vi "sutter driver track targ.vi"() -> ()   [LabVIEW 2016]
uses:
  <vilib>/userdefined/High Color/IMAQdx.ctl
  <vilib>/Instr/_visa.llb/VISA Configure Serial Port (Instr).vi
  <vilib>/vision/driver/NI_Vision_Acquisition_Software.lvlib
panel:
  out "Numeric 2":i32
  out "appended array":sgl[][](array[numeric])
  out "output array":dbl[](array[numeric])
  out "error out":errorcluster
  in  "stop":bool
  out "Send Position":dbl[](array[numeric])
  out "Curent Position":dbl[](array[numeric])
  out "Numeric":i32
  in  "VISA resource name":refnum<visa-resource-name>
  out "Pos error":sgl[](array[numeric])
  out "Injector Pos":sgl[](array[numeric])
  out "Coordinates":i32[](array[numeric])
  out "Image":T1(plugin-control)
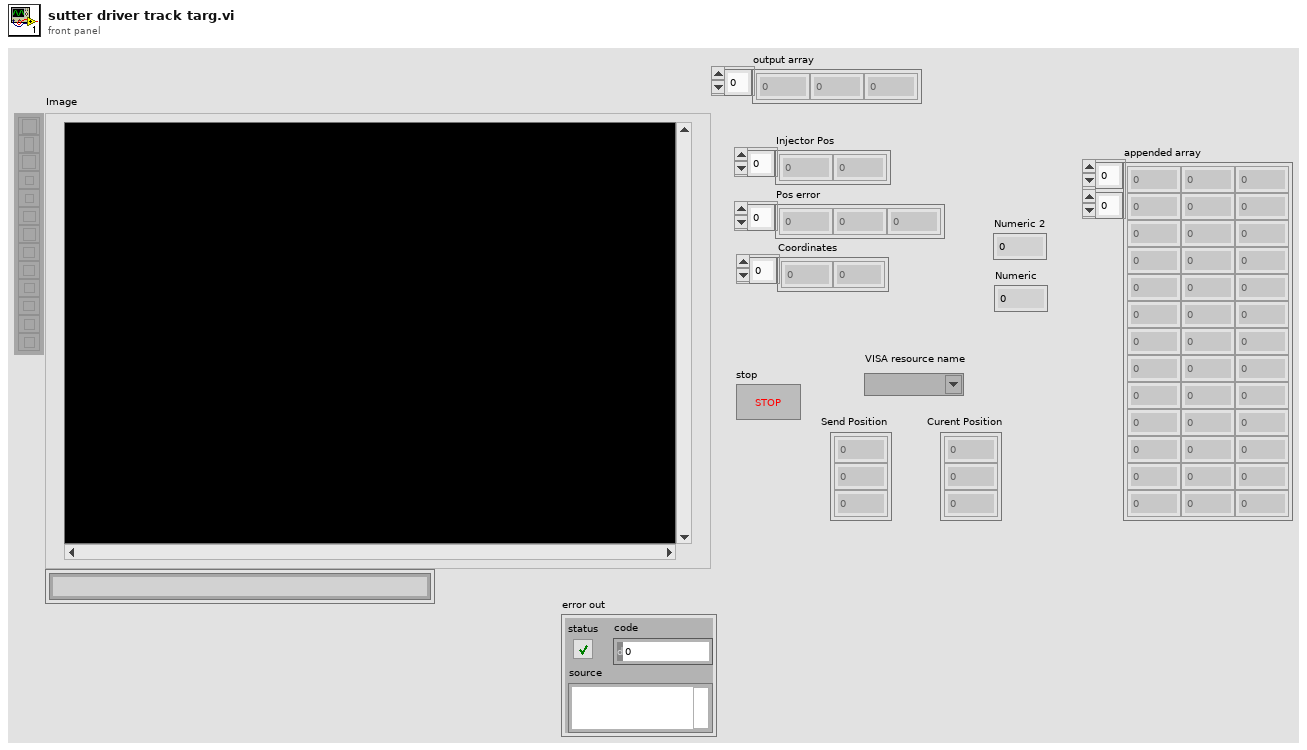
[diagram p1: front panel]
types:
  T1 = typedef "IMAQ Image.ctl" = refnum<image>
  T2 = typedef "IMAQdx.ctl" = refnum<k21>
  T3 = typedef "Image Type" = u32
  T4 = cluster{"Left":i32, "Top":i32, "Right":i32, "Bottom":i32}
  T5 = cluster{"Position":cluster{"x":sgl, "y":sgl}, "Angle":sgl, "Scale":sgl, "Score":sgl, "Bounding Box":cluster{"x":sgl, "y":sgl}[]}[]
  T6 = cluster{"Position":cluster{"x":sgl, "y":sgl}, "Angle":sgl, "Scale":sgl, "Score":sgl, "Bounding Box":cluster{"x":sgl, "y":sgl}[]}
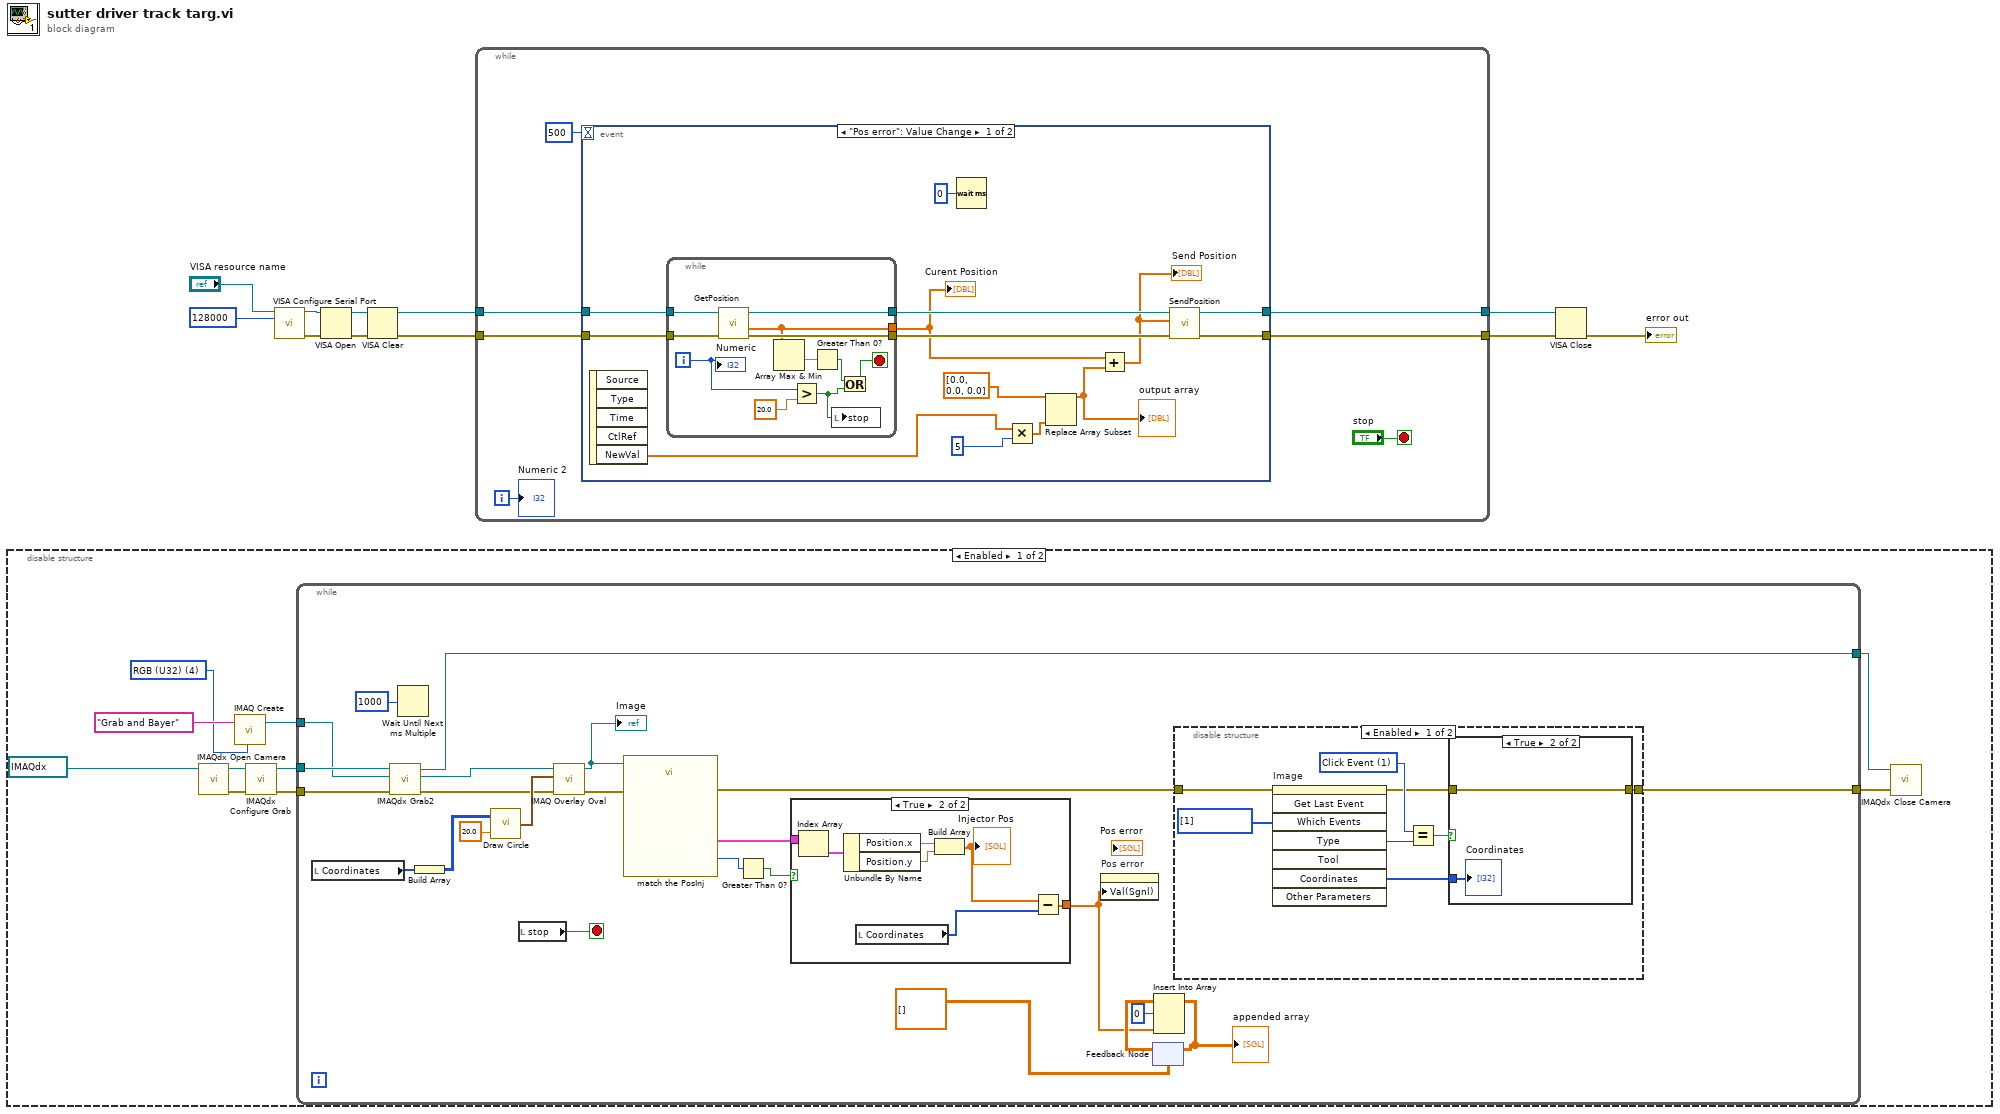
[diagram p0: block diagram]
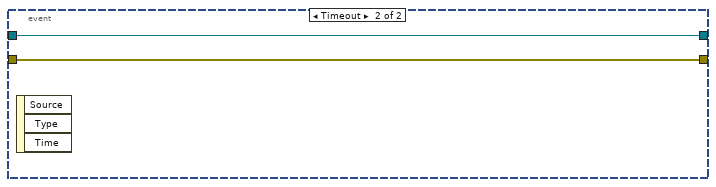
[diagram p2: hidden frame]
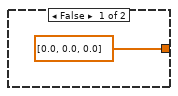
[diagram p3: hidden frame]
diagram:
  n1 = disable-structure shown="Enabled" {
    frame Enabled {
      w14 = T3 4 items=["Grayscale (U8)", "Grayscale (I16)", "Grayscale (SGL)", "Complex (CSG)", "RGB (U32)", "HSL (U32)", "RGB (U64)", "Grayscale (U16)"] ("Image Type")
      n2 = call <vilib>:"IMAQdx Open Camera.vi"("Session In"=T2 "cam1") -> ("error out"=w17:errorcluster, "Session Out"=w18:T2)  [unwired: 2 in, 7 out]
      n3 = call "IMAQ Create"("Image Name"="Grab and Bayer", "Image Type"=w14) -> ("New Image"=w15:T1)  [unwired: 2 in, 2 out]
      n4 = call <vilib>:"IMAQdx Configure Grab.vi"("error in"=w17, "Session In"=w18) -> ("error out"=w20:errorcluster, "Session Out"=w19:T2)  [unwired: 8 out]
      n5 = while {
        tunnel: w15 -> [w43]
        tunnel: w20 -> [w44]
        tunnel: w19 -> [w45]
        tunnel: [w34] -> w13
        tunnel: [w29] -> w12
        stop <- w41 stop-if-true
        n6 = local read "Coordinates"() -> (w40:i32[])
        n7 = call <vilib>:"IMAQdx Grab2.vi"("error in"=w44, "Image In"=w43, "Session In"=w45) -> ("error out"=w35:errorcluster, "Image Out"=w37:T1, "Session Out"=w34:T2)  [unwired: 5 in, 1 out]
        n8 = Wait Until Next ms Multiple(millisecond multiple=u32 1000) -> ()  [unwired: 1 out]
        n9 = Build Array(w40) -> (w39:i32[][])
        n10 = call "Draw Circle.vi"("radius"=20.0, "Pos XY"=w39) -> ("Bound out"=w36:T4)
        n11 = local read "stop"() -> (w41:bool)
        n12 = call "IMAQ Overlay Oval"("error in (no error)"=w35, "Bounding Rectangle"=w36, "Image"=w37) -> ("error out"=w31:errorcluster, "Image Out"=w32:T1)  [unwired: 7 in]
        "Image" <- w32
        n13 = call "match the PosInj"("Image In"=w32, "error in"=w31) -> ("Matches (Pattern Matching 1)"=w33:T5, "Number of Matches (Pattern Matching 1)"=w28:i32, "error out"=w30:errorcluster)  [unwired: 22 in, 1 out]
        n14 = Greater Than 0?(x=w28) -> (x > 0?=w27:bool)
        n15 = case shown="True" w27 {
          tunnel: w33 -> [_ w53]
          tunnel: [sgl[] [0.0, 0.0, 0.0] w47] -> w22
          frame False {
          }
          frame True {
            n16 = Index Array(array=w53) -> (element=w50:T6)  [unwired: 1 in]
            n17 = Unbundle By Name(w50) -> ("Position.x"=w52:sgl, "Position.y"=w51:sgl)
            n18 = local read "Coordinates"() -> (w48:i32[])
            n19 = Build Array(w52, w51) -> (w49:sgl[])
            "Injector Pos" <- w49
            n20 = Subtract(x=w49, y=w48) -> (x-y=w47:sgl[])
          }
        }
        n21 = property on="Pos error" class="Arr (strict)"("Val(Sgnl)"=w22) -> ()  [unwired: 2 in, 2 out]
        n22 = feedback #1(dbl[][] []) -> (w24:dbl[][])
        n23 = Insert Into Array(array=w24, index (row)=0, new element=w22) -> (w26:dbl[][])  [unwired: 1 in]
        "appended array" <- w26
        n24 = feedback-in #1(w26) -> ()
        n25 = disable-structure shown="Enabled" {
          disable-tunnel: [w55 _] -> w29
          disable-tunnel: w30 -> [w54 _]
          frame Enabled {
            w59 = 1 items=["No Event"=0, "Click Event"=1, "Draw Event"=2, "Size Event"=4, "Scroll Event"=5, "Double Click Event"=8]
            w60 = i32[] [1] items=["No Event"=0, "Click Event"=1, "Draw Event"=2, "Size Event"=4, "Scroll Event"=5, "Double Click Event"=8] ("Which Events")
            n26 = invoke on="Image" class="ImageControl" method="Get Last Event"(error in=w54, "Which Events"=w60) -> (error out=w56:errorcluster, "Type"=w58:i32, "Coordinates"=w61:i32[])  [unwired: 6 in, 5 out]
            n27 = Equal?(x=w59, y=w58) -> (x = y?=w57:bool)
            n28 = case shown="True" w57 {
              tunnel: w61 -> [_ w64]
              tunnel: w56 -> [w62 w63]
              tunnel: [w62 w63] -> w55
              frame False {
              }
              frame True {
                "Coordinates" <- w64
              }
            }
          }
          frame Disabled {
          }
        }
      }
      n29 = call <vilib>:"IMAQdx Close Camera.vi"("error in"=w12, "Session In"=w13) -> ()  [unwired: 9 in, 1 out]
    }
    frame Disabled {
    }
  }
  n30 = call-poly "VISA Configure Serial Port"("VISA resource name"="VISA resource name", "baud rate (9600)"=u32 128000) -> ("VISA resource name out"=w9:refnum<visa-resource-name>, "error out"=w8:errorcluster)  [unwired: 12 in]
  n31 = VISA Open(error in (no error)=w8, VISA resource name=w9) -> (VISA resource name=w4:refnum<visa-resource-name>, error out=w3:errorcluster)  [unwired: 3 in]
  n32 = VISA Clear(VISA resource name=w4, error in (no error)=w3) -> (VISA resource name out=w2:refnum<visa-resource-name>, error out=w1:errorcluster)
  n33 = while {
    tunnel: w1 -> [w69]
    tunnel: [w70] -> w6
    tunnel: w2 -> [w68]
    tunnel: [w71] -> w7
    i -> [w66]
    stop <- "stop" stop-if-true
    n34 = event shown="[0] \"Pos error\": Value Change" {
      selector: _ -> [_ _]
      dyn-events: _ -> [_ _]
      timeout: 500 -> [_ _]
      tunnel: [w85 w97] -> w71
      tunnel: [w84 w98] -> w70
      tunnel: w68 -> [w83 w97]
      tunnel: w69 -> [w80 w98]
      event "Pos error": Value Change {
        n35 = event-data() -> ("NewVal"=w73:sgl[])  [unwired: 1 in, 4 out]
        n36 = while {
          tunnel: [w92] -> w77
          tunnel: w83 -> [w95]
          tunnel: [w94] -> w82
          tunnel: w80 -> [w96]
          tunnel: [w93] -> w81
          i -> [w90]
          stop <- w87 stop-if-true
          n37 = call "GetPosition.vi"("error in"=w96, "VISA resource name in"=w95) -> ("error out"=w93:errorcluster, "Position XYZ"=w92:dbl[], "VISA resource name out"=w94:refnum<visa-resource-name>)  [unwired: 3 in, 1 out]
          n38 = Array Max & Min(array=w92) -> (min value=w89:dbl)  [unwired: 3 out]
          n39 = Greater?(x=w90, y=20.0) -> (0:w86:bool)
          n40 = Greater Than 0?(x=w89) -> (x > 0?=w88:bool)
          n41 = local write "stop"(w86) -> ()
          n42 = Or(x=w88, y=w86) -> (x .or. y?=w87:bool)
          "Numeric" <- w90
        }
        "Curent Position" <- w77
        n43 = Wait (ms)(milliseconds to wait=u32 0) -> ()  [unwired: 1 out]
        n44 = Multiply(x=w73, y=5 ("number: 0 to 1")) -> (x*y=w76:sgl[])
        n45 = Replace Array Subset(array=dbl[] [0.0, 0.0, 0.0], new element=w76) -> (w74:dbl[])  [unwired: 1 in]
        "output array" <- w74
        n46 = Add(x=w77, y=w74) -> (x+y=w78:dbl[])
        "Send Position" <- w78
        n47 = call "SendPosition.vi"("error in"=w81, "Motor Position"=w78, "VISA resource In"=w82) -> ("error out"=w84:errorcluster, "VISA resource name out"=w85:refnum<visa-resource-name>)  [unwired: 5 in]
      }
      event Timeout {
        n48 = event-data() -> ()  [unwired: 1 in, 3 out]
      }
    }
    "Numeric 2" <- w66
  }
  n49 = VISA Close(VISA resource name=w7, error in (no error)=w6) -> (error out=→"error out":errorcluster)
